vi "SSC Digital Calculate Per-Instrument to Per-Site Per-Pin LUT.vi"(0 "Digital SSC In":T3[](array[typedef]), 7 "Sites":i32[](array[numeric]), 9 "Pins":string[](array[string])) -> (4 "Per-Instrument to Per-Site Per-Pin LUT":T1[](array[typedef]))   [LabVIEW 2019]
uses:
  SSC Digital/SSC Digital.ctl
  Digital 2D Location Array in a Cluster.ctl
  Digital 2D Location.ctl
  Shared SubVIs/Trim Whitespace [Inlined].vi
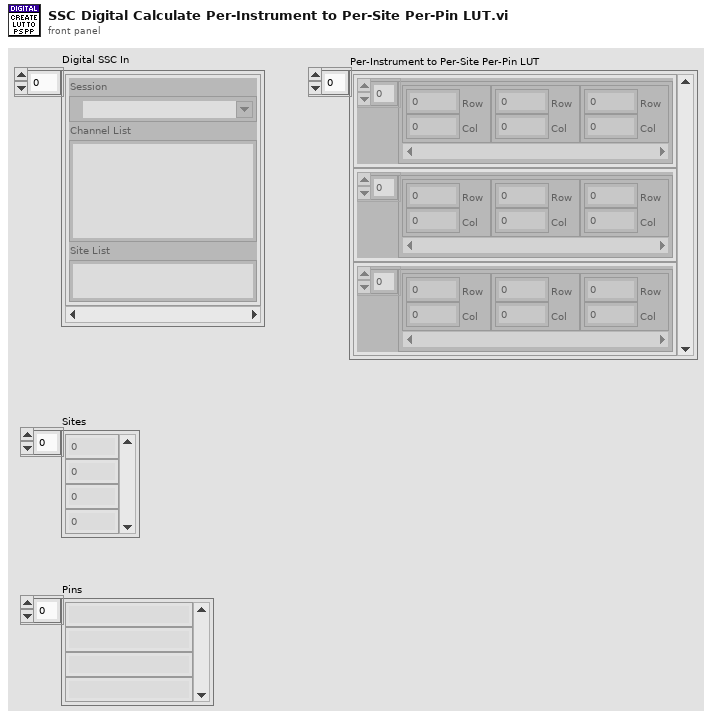
[diagram p1: front panel]
types:
  T1 = typedef "Digital 2D Location Array in a Cluster.ctl" = cluster{"Digital 2D Location Array":T2[]}
  T2 = typedef "Digital 2D Location.ctl" = cluster{"Row":i32, "Col":i32}
  T3 = typedef "SSC Digital.ctl" = cluster{"Session":refnum<k15>, "Channel List":string, "Site List":string}
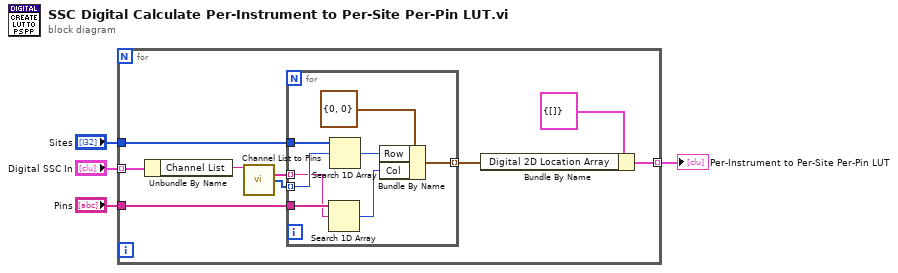
[diagram p0: block diagram]
diagram:
  n1 = for {
    tunnel: "Digital SSC In" -> [w13] mode=indexing
    tunnel: "Sites" -> [w8]
    tunnel: "Pins" -> [w9]
    tunnel: [w6] -> w1 mode=indexing
    n2 = Unbundle By Name(w13) -> ("Channel List"=w12:string)
    n3 = call "Channel List to Pins.vi"("Channel List"=w12) -> ("Pins"=w11:tag[], "Sites"=w10:i32[])  [unwired: 12 in, 1 out]
    n4 = for {
      tunnel: w11 -> [w18] mode=indexing
      tunnel: w10 -> [w20] mode=indexing
      tunnel: w9 -> [w19]
      tunnel: w8 -> [w21]
      tunnel: [w17] -> w7 mode=indexing
      n5 = Search 1D Array(1D array=w19, element=w18) -> (index of element=w15:i32)  [unwired: 1 in]
      n6 = Search 1D Array(1D array=w21, element=w20) -> (index of element=w16:i32)  [unwired: 1 in]
      n7 = Bundle By Name(cluster=T2 {"Row"=0, "Col"=0}, "Row"=w16, "Col"=w15) -> (w17:T2)
    }
    n8 = Bundle By Name(cluster=T1 {"Digital 2D Location Array"=[]} ("Digital 2D Location Array in a Cluster"), "Digital 2D Location Array"=w7) -> (w6:T1)
  }
  "Per-Instrument to Per-Site Per-Pin LUT" <- w1
